vi "Send Reset Active DTC to Main.vi"(8 "error in (no error)":errorcluster, 10 "Address":u8, 11 "Simulated Addresses LUT":variant) -> (0 "error out":errorcluster, 2 "found":bool)   [LabVIEW 2013, in "J1939 Addon Engine.lvlib"]
uses:
  J1939 Addon Engine.lvlib
  Types/Simulated Settings.ctl
  Shared/Types/Compiled Simulated Settings.ctl
  Shared/Types/Monitor Settings.ctl
  <vilib>/NI Veristand/Custom Device API/Block Data Reference.ctl
  <vilib>/NI Veristand/Custom Device API/Data Reference.ctl
  Types/DTC FIFOs.ctl
  <vilib>/NI Veristand/Custom Device API/Custom Device API.lvlib
  Shared/J1939 Addon Shared.lvlib
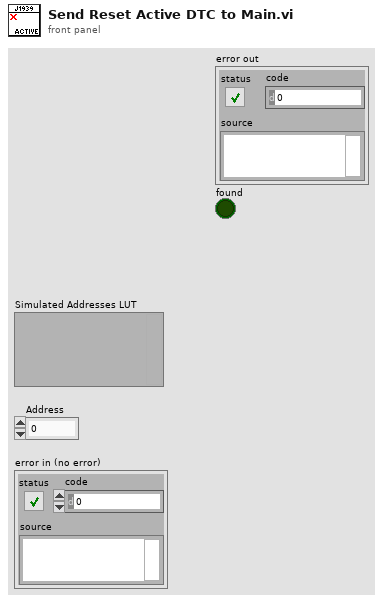
[diagram p1: front panel]
types:
  T1 = typedef "J1939 Addon Engine.lvlib/Simulated Settings.ctl" = cluster{"Simulated Addresses":T2, "FIFOs":T6}
  T2 = typedef "J1939 Addon Shared.lvlib/Compiled Simulated Settings.ctl" = cluster{"J1939 XNET Settings":T3, "DM1 Data":T4[], "DM1 Data":dbl[], "DM1 Enable?":T4[], "DM1 Enable?":dbl[], "DM2 Data":T4[], "DM2 Data":dbl[], "DM2 Enable?":T4[], "DM2 Enable?":dbl[]}
  T3 = typedef "J1939 Addon Shared.lvlib/Monitor Settings.ctl" = cluster{"J1939 Network Address":u8, "Name":u64}
  T4 = typedef "Custom Device API.lvlib/Block Data Reference.ctl" = cluster{"Data Reference":T5, "Offset":i32, "Length":i32}
  T5 = typedef "Custom Device API.lvlib/Data Reference.ctl" = i32
  T6 = typedef "J1939 Addon Engine.lvlib/DTC FIFOs.ctl" = cluster{"DM1 Data":refnum<k33>, "DM1 Enable?":refnum<k33>, "DM2 Data":refnum<k33>, "DM2 Enable?":refnum<k33>, "DM1 Reset?":refnum<k33>, "DM2 Reset?":refnum<k33>}
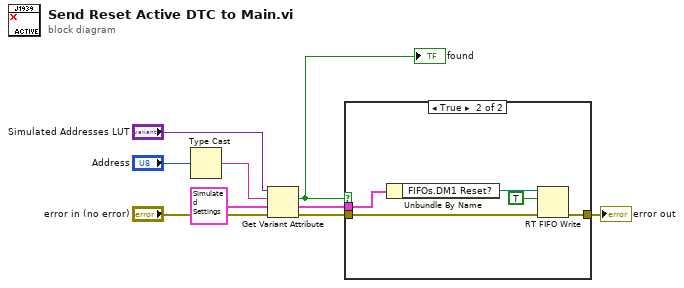
[diagram p0: block diagram]
diagram:
  n1 = Type Cast(x="Address") -> (*(type *) &x=w7:string)  [unwired: 1 in]
  n2 = Get Variant Attribute(Variant="Simulated Addresses LUT", name=w7, default value (empty Variant)=T1 {"Simulated Addresses"={"J1939 XNET Settings"={"J1939 Network Address"=0, "Name"=0}, "DM1 Data"=[], "DM1 Data"=[], "DM1 Enable?"=[], "DM1 Enable?"=[], "DM2 Data"=[], "DM2 Data"=[], "DM2 Enable?"=[], "DM2 Enable?"=[]}, "FIFOs"={"DM1 Data"=refnum, "DM1 Enable?"=refnum, "DM2 Data"=refnum, "DM2 Enable?"=refnum, "DM1 Reset?"=refnum, "DM2 Reset?"=refnum}} ("Cluster"), error in="error in (no error)") -> (found=w4:bool, value=w2:T1, error out=w3:errorcluster)  [unwired: 1 out]
  "found" <- w4
  n3 = case shown="True" w4 {
    tunnel: w3 -> [w10 w13]
    tunnel: w2 -> [_ w15]
    tunnel: [w10 w11] -> w1
    frame False {
    }
    frame True {
      n4 = Unbundle By Name(w15) -> ("FIFOs.DM1 Reset?"=w14:refnum<k33>)
      n5 = RT FIFO Write(0:w14, 1:TRUE ("element"), 3:w13) -> (11:w11:errorcluster)  [unwired: 2 in, 3 out]
    }
  }
  "error out" <- w1
